vi "Test Rotation.vi"() -> ()   [LabVIEW 2017]
panel:
  out "Numeric":i32
  in  "Array 2":i32[][](array[numeric])=[[1, 0, 0, 0], [1, 0, 0, 0], [1, 0, 0, 0], [1, 0, 0, 0]]
  in  "stop":bool
  in  "Rotate":bool
  out "Array":i32[][](array[numeric])
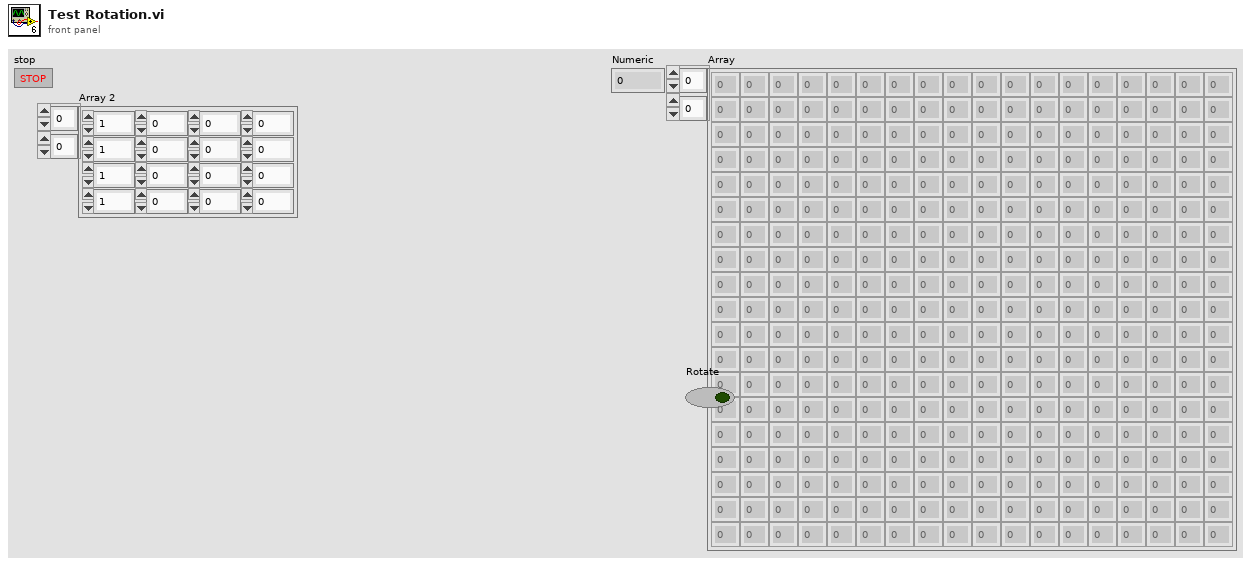
[diagram p1: front panel]
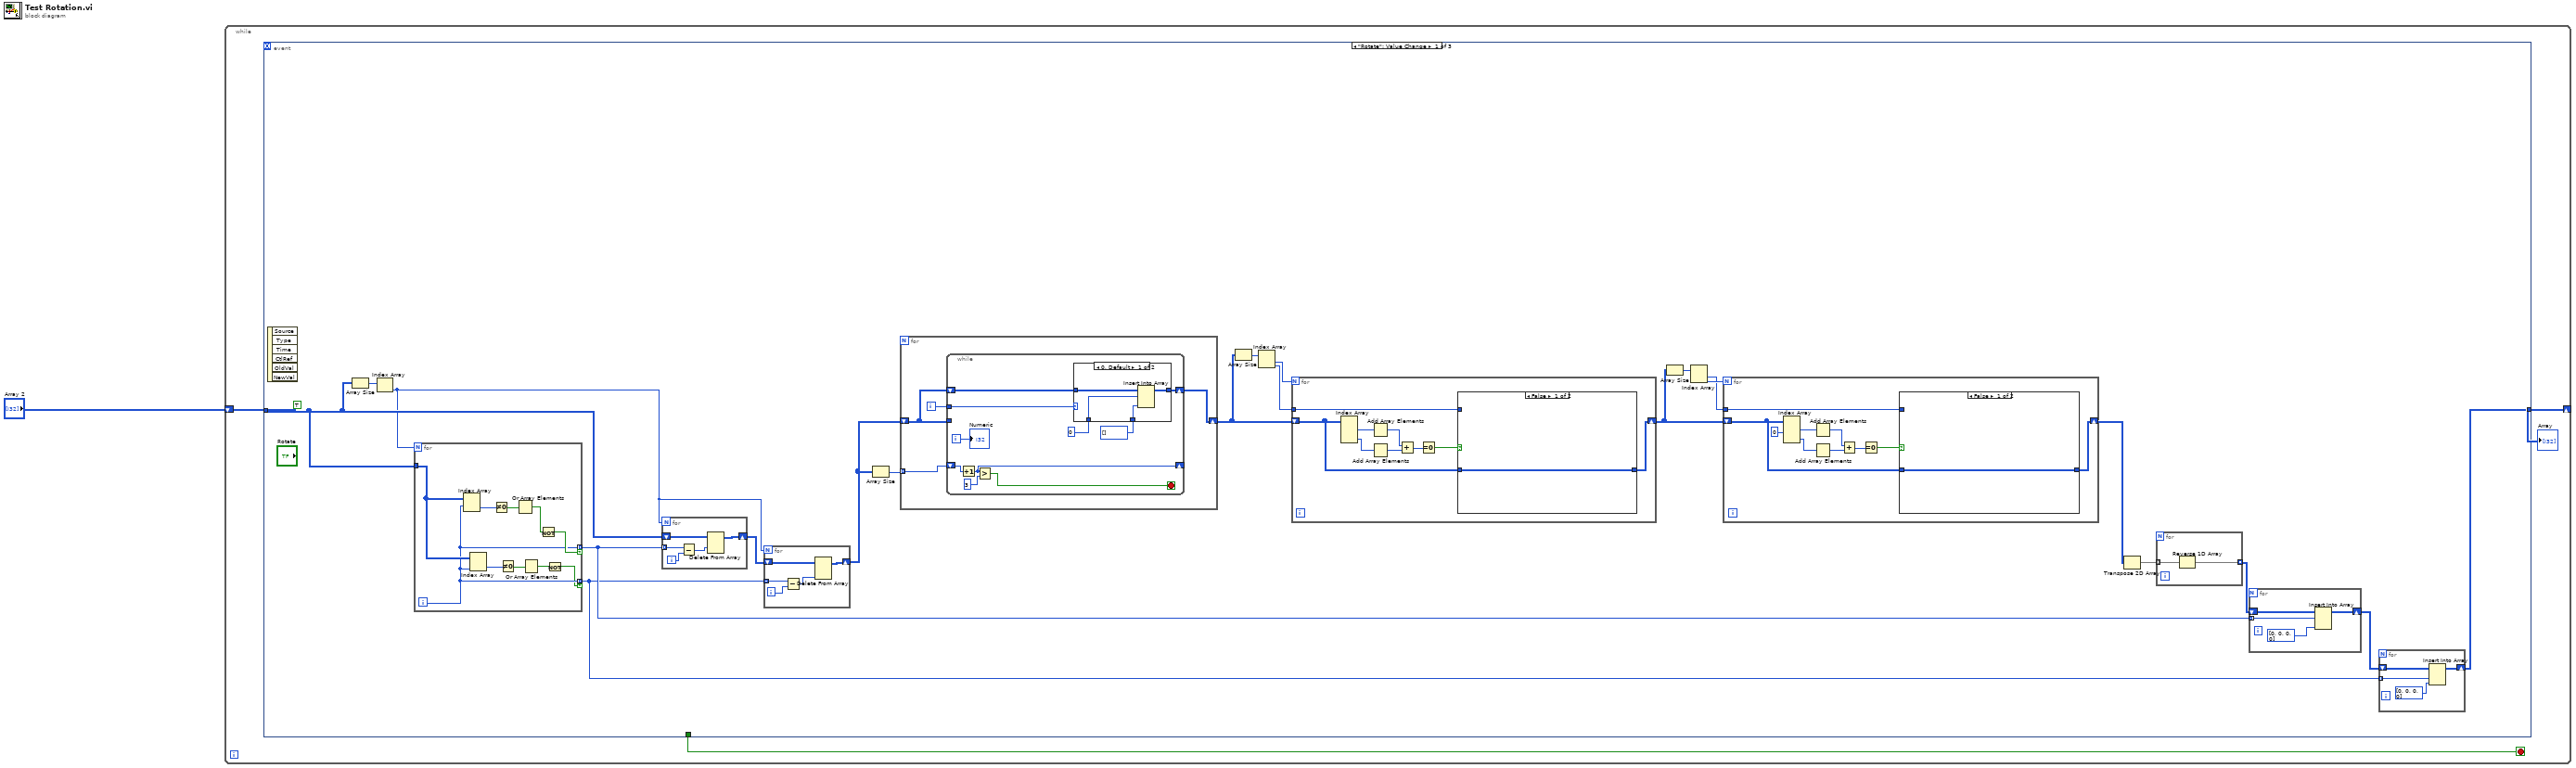
[diagram p0: block diagram]
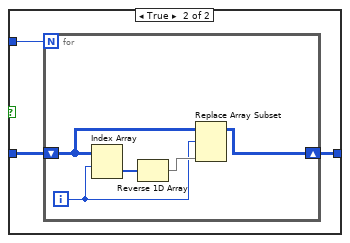
[diagram p2: hidden frame]
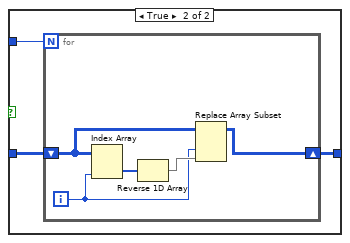
[diagram p3: hidden frame]
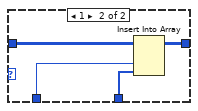
[diagram p4: hidden frame]
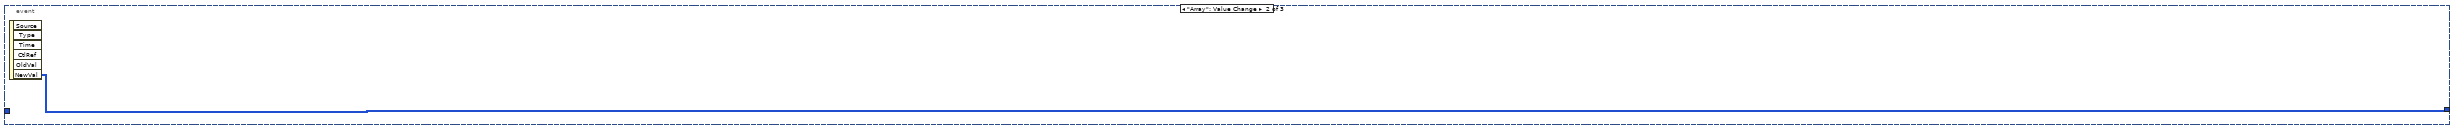
[diagram p5: hidden frame]
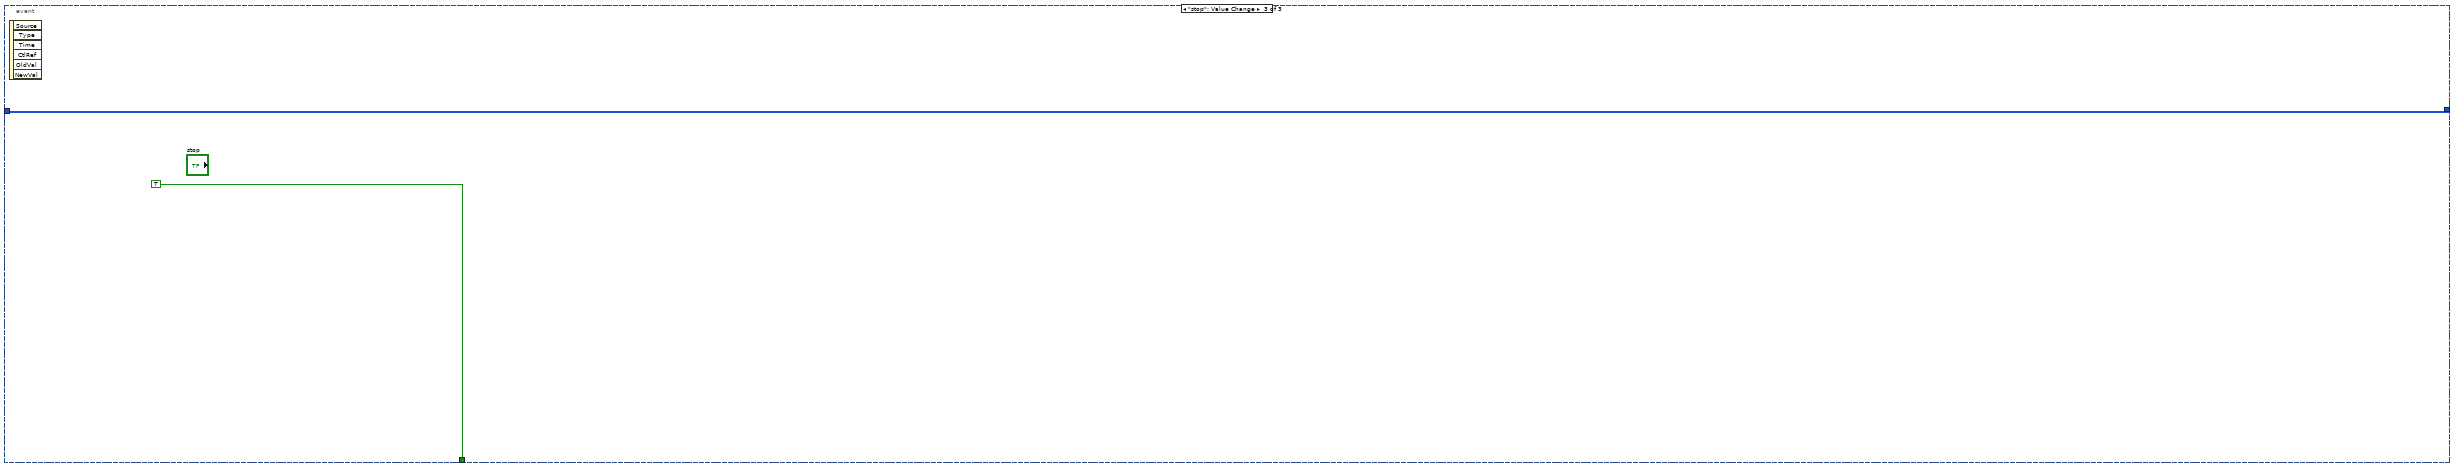
[diagram p6: hidden frame]
diagram:
  n1 = while {
    shift-right: [w2] -> _
    shift-left: "Array 2" -> [w4]
    stop <- w3 stop-if-true
    n2 = event shown="[0] \"Rotate\": Value Change" {
      selector: _ -> [_ _ _]
      dyn-events: _ -> [_ _ _]
      timeout: _ -> [_ _ _]
      tunnel: w4 -> [w18 _ w116]
      tunnel: [w19 w115 w116] -> w2
      tunnel: [_ _ TRUE ("stop")] -> w3
      event "Rotate": Value Change {
        (unwired) TRUE
        n3 = event-data() -> ()  [unwired: 1 in, 6 out]
        n4 = Array Size(array=w18) -> (size(s)=w17:i32[])
        n5 = Index Array(array=w17) -> (element=w16:i32)  [unwired: 1 in]
        n6 = for {
          N: w16 -> [_]
          tunnel: [w106] -> w21 mode=indexing if=w111
          tunnel: [w106] -> w20 mode=indexing if=w105
          tunnel: w18 -> [w107]
          i -> [w106]
          n7 = Index Array(array=w107, index (row)=w106) -> (element=w114:i32[])  [unwired: 1 in]
          n8 = Index Array(array=w107, index (col)=w106) -> (element=w110:i32[])  [unwired: 1 in]
          n9 = Not Equal To 0?(x=w114) -> (x != 0?=w113:bool[])
          n10 = Not Equal To 0?(x=w110) -> (x != 0?=w109:bool[])
          n11 = Or Array Elements(Boolean array=w113) -> (logical OR=w112:bool)
          n12 = Or Array Elements(Boolean array=w109) -> (logical OR=w108:bool)
          n13 = Not(x=w112) -> (.not. x?=w111:bool)
          n14 = Not(x=w108) -> (.not. x?=w105:bool)
        }
        n15 = for {
          N: w16 -> [_]
          tunnel: w21 -> [w101] mode=indexing
          shift-right: [w103] -> w25
          shift-left: w18 -> [w104]
          i -> [w102]
          n16 = Subtract(x=w101, y=w102) -> (x-y=w100:i32)
          n17 = Delete From Array(array=w104, index (row)=w100) -> (array with subset deleted=w103:i32[][])  [unwired: 2 in, 1 out]
        }
        n18 = for {
          N: w16 -> [_]
          tunnel: w20 -> [w97] mode=indexing
          shift-right: [w98] -> w14
          shift-left: w25 -> [w99]
          i -> [w96]
          n19 = Subtract(x=w97, y=w96) -> (x-y=w95:i32)
          n20 = Delete From Array(array=w99, index (col)=w95) -> (array with subset deleted=w98:i32[][])  [unwired: 2 in, 1 out]
        }
        n21 = Array Size(array=w14) -> (size(s)=w15:i32[])
        n22 = for {
          tunnel: w15 -> [w66] mode=indexing
          shift-right: [w64] -> w13
          shift-left: w14 -> [w63]
          i -> [w65]
          n23 = while {
            shift-right: [w69] -> _
            shift-left: w66 -> [w70]
            tunnel: w63 -> [_]
            tunnel: w65 -> [w74]
            shift-right: [w72] -> w64
            shift-left: w63 -> [w71]
            i -> [w67]
            stop <- w75 stop-if-true
            n24 = Increment(x=w70) -> (x+1=w69:i32)
            n25 = Greater?(x=w69, y=3) -> (0:w75:bool)
            n26 = case shown="0, Default" w74 {
              tunnel: w71 -> [w80 w84]
              tunnel: i32[] [] ("new element/subarray") -> [w79 w83]
              tunnel: [w78 w82] -> w72
              tunnel: 0 -> [w77 w81]
              frame 0, Default {
                n27 = Insert Into Array(array=w80, index (row)=w77, new element=w79) -> (w78:i32[][])  [unwired: 1 in]
              }
              frame 1 {
                n28 = Insert Into Array(array=w84, index (col)=w81, new element=w83) -> (w82:i32[][])  [unwired: 1 in]
              }
            }
            "Numeric" <- w67
          }
        }
        n29 = Array Size(array=w13) -> (size(s)=w12:i32[])
        n30 = Index Array(array=w12) -> (element #1=w11:i32, element #2=w10:i32)  [unwired: 2 in]
        n31 = for {
          N: w11 -> [_]
          tunnel: w10 -> [w47]
          shift-right: [w45] -> w8
          shift-left: w13 -> [w48]
          n32 = Index Array(array=w48) -> (element #1=w53:i32[], element #2=w52:i32[])  [unwired: 4 in]
          n33 = Add Array Elements(numeric array=w53) -> (sum=w50:i32)
          n34 = Add Array Elements(numeric array=w52) -> (sum=w51:i32)
          n35 = Add(x=w50, y=w51) -> (x+y=w49:i32)
          n36 = Equal To 0?(x=w49) -> (x = 0?=w46:bool)
          n37 = case shown="False" w46 {
            tunnel: w48 -> [w54 w57]
            tunnel: w47 -> [_ w56]
            tunnel: [w54 w55] -> w45
            frame False {
            }
            frame True {
              n38 = for {
                N: w56 -> [_]
                shift-right: [w58] -> w55
                shift-left: w57 -> [w60]
                i -> [w59]
                n39 = Index Array(array=w60, index (col)=w59) -> (element=w62:i32[])  [unwired: 1 in]
                n40 = Reverse 1D Array(array=w62) -> (reversed array=w61:i32[])
                n41 = Replace Array Subset(array=w60, new element=w61, index (col)=w59) -> (w58:i32[][])  [unwired: 1 in]
              }
            }
          }
        }
        n42 = Array Size(array=w8) -> (size(s)=w9:i32[])
        n43 = Index Array(array=w9) -> (element #1=w6:i32, element #2=w7:i32)  [unwired: 2 in]
        n44 = for {
          N: w7 -> [_]
          tunnel: w6 -> [w29]
          shift-right: [w27] -> w5
          shift-left: w8 -> [w30]
          n45 = Index Array(array=w30, index (col) #1=0 ("disabled index (col)")) -> (element #1=w35:i32[], element #2=w34:i32[])  [unwired: 3 in]
          n46 = Add Array Elements(numeric array=w35) -> (sum=w32:i32)
          n47 = Add Array Elements(numeric array=w34) -> (sum=w33:i32)
          n48 = Add(x=w32, y=w33) -> (x+y=w31:i32)
          n49 = Equal To 0?(x=w31) -> (x = 0?=w28:bool)
          n50 = case shown="False" w28 {
            tunnel: w30 -> [w36 w39]
            tunnel: w29 -> [_ w38]
            tunnel: [w36 w37] -> w27
            frame False {
            }
            frame True {
              n51 = for {
                N: w38 -> [_]
                shift-right: [w41] -> w37
                shift-left: w39 -> [w42]
                i -> [w40]
                n52 = Index Array(array=w42, index (row)=w40) -> (element=w44:i32[])  [unwired: 1 in]
                n53 = Reverse 1D Array(array=w44) -> (reversed array=w43:i32[])
                n54 = Replace Array Subset(array=w42, new element=w43, index (row)=w40) -> (w41:i32[][])  [unwired: 1 in]
              }
            }
          }
        }
        n55 = Transpose 2D Array(2D array=w5) -> (transposed array=w24:i32[][])
        n56 = for {
          tunnel: w24 -> [w94] mode=indexing
          tunnel: [w93] -> w22 mode=indexing
          n57 = Reverse 1D Array(array=w94) -> (reversed array=w93:i32[])
        }
        n58 = for {
          tunnel: w21 -> [w90] mode=indexing
          shift-right: [w91] -> w23
          shift-left: w22 -> [w92]
          n59 = Insert Into Array(array=w92, index (row)=w90, new element=i32[] [0, 0, 0, 0] ("new element/subarray")) -> (w91:i32[][])  [unwired: 1 in]
        }
        n60 = for {
          tunnel: w20 -> [w86] mode=indexing
          shift-right: [w87] -> w19
          shift-left: w23 -> [w88]
          n61 = Insert Into Array(array=w88, index (col)=w86, new element=i32[] [0, 0, 0, 0] ("new element/subarray")) -> (w87:i32[][])  [unwired: 1 in]
        }
      }
      event "Array": Value Change {
        n62 = event-data() -> ("NewVal"=w115:i32[][])  [unwired: 1 in, 5 out]
      }
      event "stop": Value Change {
        n63 = event-data() -> ()  [unwired: 1 in, 6 out]
      }
    }
    "Array" <- w2
  }
